vi "VXM-Jog.vi"(8 "error in (no error)":errorcluster, 9 "Direction":i32=1, 10 "mmWave Axis":T2="BS1", 11 "Message que":T1) -> (0 "error out":errorcluster)   [LabVIEW 2019]
uses:
  mmWaveAxis.ctl
  Support/MessageQue/MessageQue.ctl
  Support/MessageQue/MessageCluster.ctl
  Support/MessageQue/MessageQue.lvlib
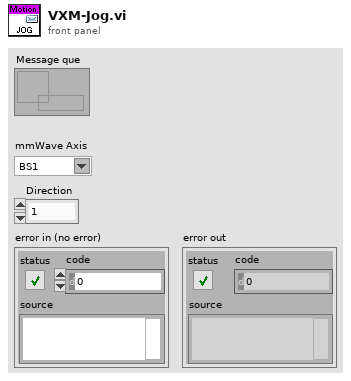
[diagram p1: front panel]
types:
  T1 = typedef "MessageQue.lvlib/MessageQue.ctl" = refnum<queue>
  T2 = typedef "mmWaveAxis.ctl" = string
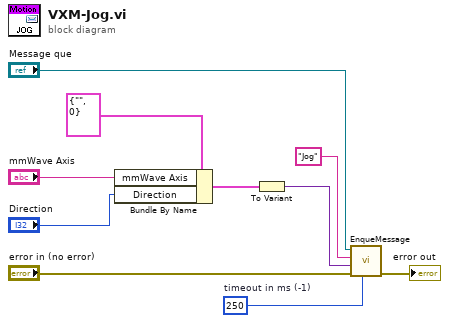
[diagram p0: block diagram]
diagram:
  w9 = 250  # timeout in ms (-1)
  n1 = Bundle By Name(cluster=cluster{"mmWave Axis":T2, "Direction":i32} {"mmWave Axis"="", "Direction"=0} ("output cluster"), "mmWave Axis"="mmWave Axis", "Direction"="Direction") -> (w2:cluster{"mmWave Axis":T2, "Direction":i32})
  n2 = To Variant(anything=w2) -> (Variant=w10:variant)
  n3 = call "EnqueMessage.vi"("timeout in ms (-1)"=w9, "error in"="error in (no error)", "Message Payload"=w10, "Message Command"="Jog", "Message que"="Message que") -> ("error out"=→"error out":errorcluster)  [unwired: 5 in, 1 out]
